vi "main.vi"() -> ()   [LabVIEW 2020]
uses:
  PCANBasic/eX/CTLs/TPCANHandle-Channel_eX.ctl
  PCANBasic/eX/CTLs/TPCANHandle-Bitrate_eX.ctl
  PCANBasic/eX/CTLs/CAN MSG_eX.ctl
  PCANBasic/eX/CTLs/CAN ErrorTypes_eX.ctl
  PCANBasic/PCANBasic_eX.lvlib
panel:
  out "error out":errorcluster
  out "Rotary Init REPONSE ?":bool
  in  "stop":bool
  in  "SetBrightness":bool
  in  "Brightness \n(0xFE = OFF, 0xFD=MAX)":u8=253 format="%02x"
  in  "TPCANHandle-Bitrate":T1=enum."500 KBit/s"
  in  "TPCANHandle-Channel":T2
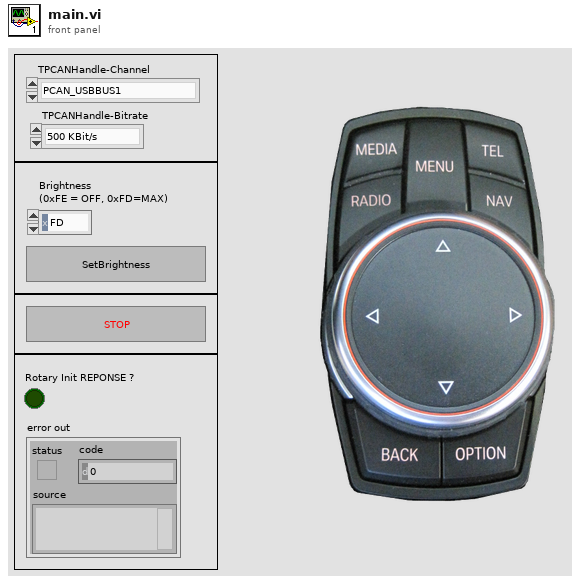
[diagram p1: front panel]
types:
  T1 = typedef "PCANBasic_eX.lvlib/TPCANHandle-Bitrate_eX.ctl" = enum16{"1 Mbit/s", "800 KBit/s", "500 KBit/s", "250 KBit/s", "125 KBit/s", "100 KBit/s"}
  T2 = typedef "PCANBasic_eX.lvlib/TPCANHandle-Channel_eX.ctl" = enum16{"PCAN_USBBUS1", "PCAN_USBBUS2"}
  T3 = typedef "PCANBasic_eX.lvlib/CAN MSG_eX.ctl" = cluster{"ID":u32, "MSGTYPE":u8, "LEN":u8, "DATA[0]":u8, "DATA[1]":u8, "DATA[2]":u8, "DATA[3]":u8, "DATA[4]":u8, "DATA[5]":u8, "DATA[6]":u8, "DATA[7]":u8}
  T4 = typedef "PCANBasic_eX.lvlib/CAN ErrorTypes_eX.ctl" = enum16{"ERROR_INIT", "ERROR_SEND_MSG", "ERROR_RECV_MSG", "ERROR_RESET", "ERROR_FILTER", "ERROR_UNINIT"}
  T5 = typedef "PCANBasic_eX.lvlib/CAN Timestamp_eX.ctl" = cluster{"millis":u32, "millis_overflow":u16, "micros":u16}
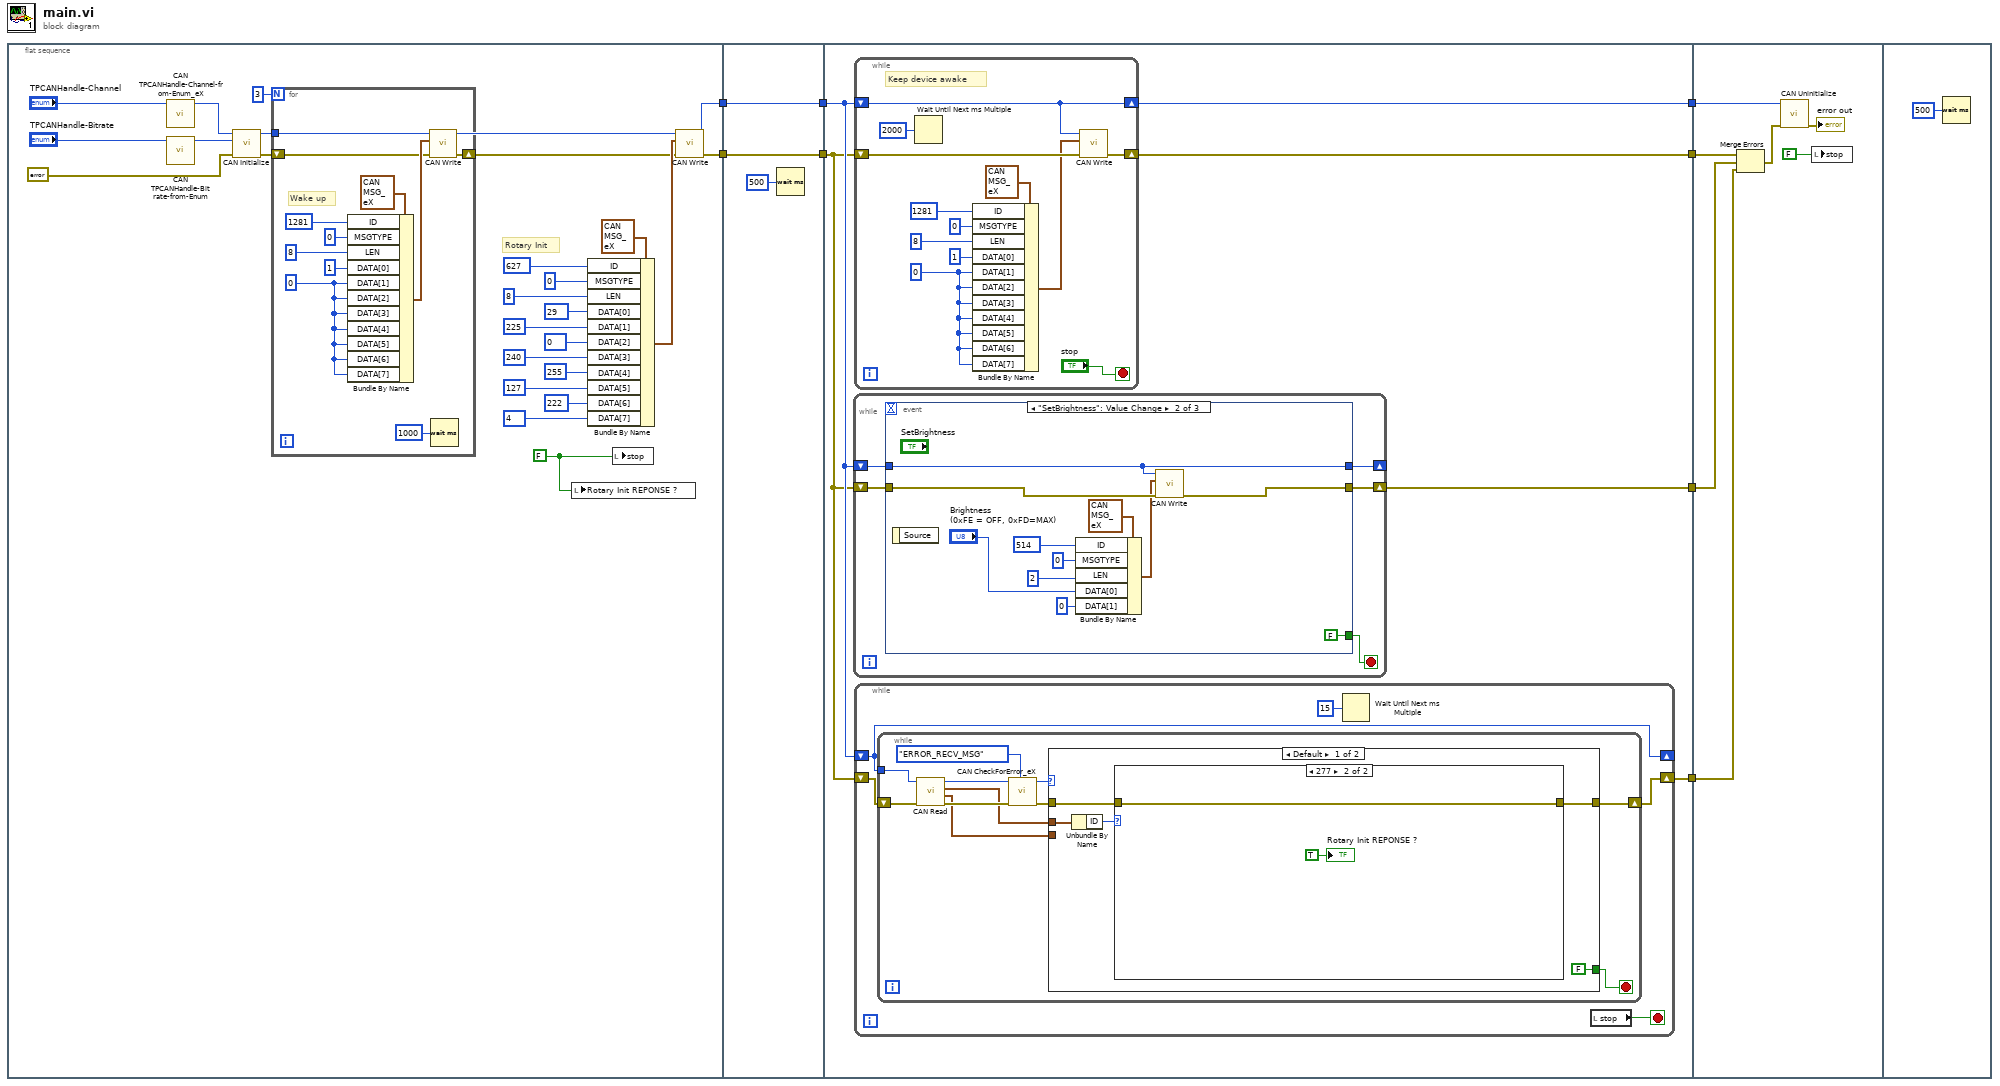
[diagram p0: block diagram]
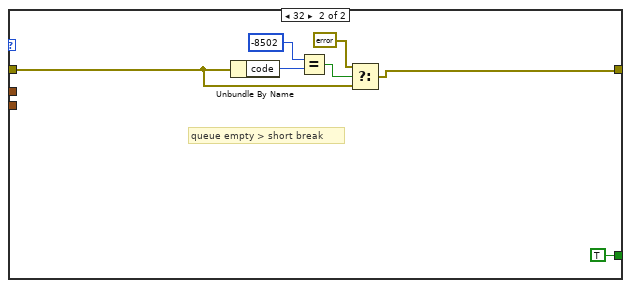
[diagram p3: hidden frame]
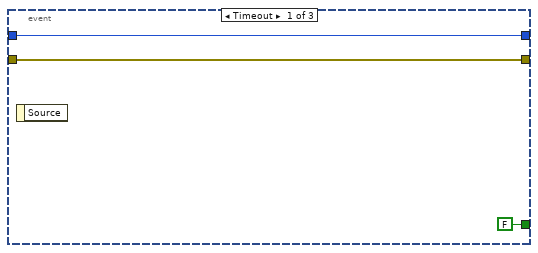
[diagram p4: hidden frame]
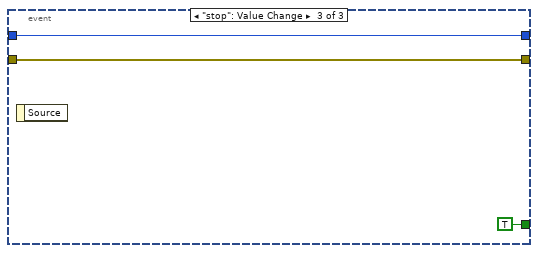
[diagram p5: hidden frame]
diagram:
  n1 = flat-sequence {
    tunnel: [w26] -> w8
    tunnel: [w25] -> w6
    tunnel: w8 -> [w45]
    tunnel: [w45] -> w7
    tunnel: w6 -> [w44]
    tunnel: [w44] -> w5
    tunnel: w7 -> [w50]
    tunnel: w5 -> [w51]
    tunnel: [w49] -> w4
    tunnel: [w48] -> w3
    tunnel: [w47] -> w2
    tunnel: [w46] -> w1
    tunnel: w4 -> [w123]
    tunnel: w3 -> [w122]
    tunnel: w2 -> [w121]
    tunnel: w1 -> [w119]
    frame #0 {
      w11 = FALSE ("stop")
      # "Rotary Init"
      n2 = call "CAN TPCANHandle-Channel-from-Enum_eX.vi"("TPCANHandle-Channel"="TPCANHandle-Channel") -> ("Channel"=w25:u16)  [unwired: 10 in]
      n3 = call "CAN TPCANHandle-Bitrate-from-Enum.vi"("TPCANHandle-Bitrate"="TPCANHandle-Bitrate") -> ("Btr0Btr1"=w31:u16)  [unwired: 10 in]
      n4 = call "CAN Initialize.vi"("error in (no error)"=errorcluster {"status"=FALSE, "code"=0, "source"=""}, "Btr0Btr1"=w31, "Channel"=w25) -> ("error out"=w27:errorcluster)  [unwired: 7 in, 1 out]
      n5 = for {
        N: 3 -> [_]
        tunnel: w25 -> [w34]
        shift-right: [w33] -> w10
        shift-left: w27 -> [w35]
        w42 = u8 0 ("DATA[1]")
        # "Wake up"
        n6 = Bundle By Name(cluster=T3 {"ID"=261, "MSGTYPE"=0, "LEN"=8, "DATA[0]"=37, "DATA[1]"=80, "DATA[2]"=37, "DATA[3]"=80, "DATA[4]"=37, "DATA[5]"=80, "DATA[6]"=37, "DATA[7]"=80} ("MessageBuffer"), "ID"=u32 1281, "MSGTYPE"=u8 0, "LEN"=u8 8, "DATA[0]"=u8 1, "DATA[1]"=w42, "DATA[2]"=w42, "DATA[3]"=w42, "DATA[4]"=w42, "DATA[5]"=w42, "DATA[6]"=w42, "DATA[7]"=w42) -> (w37:T3)
        n7 = call "CAN Write.vi"("error in (no error)"=w35, "MessageBuffer"=w37, "Channel"=w34) -> ("error out"=w33:errorcluster)  [unwired: 6 in, 2 out]
        n8 = Wait (ms)(milliseconds to wait=u32 1000) -> ()  [unwired: 1 out]
      }
      n9 = local write "Rotary Init REPONSE ?"(w11) -> ()
      n10 = Bundle By Name(cluster=T3 {"ID"=261, "MSGTYPE"=0, "LEN"=8, "DATA[0]"=37, "DATA[1]"=80, "DATA[2]"=37, "DATA[3]"=80, "DATA[4]"=37, "DATA[5]"=80, "DATA[6]"=37, "DATA[7]"=80} ("MessageBuffer"), "ID"=u32 627, "MSGTYPE"=u8 0, "LEN"=u8 8, "DATA[0]"=u8 29, "DATA[1]"=u8 225 ("DATA[0]"), "DATA[2]"=u8 0 ("DATA[0]"), "DATA[3]"=u8 240 ("DATA[0]"), "DATA[4]"=u8 255 ("DATA[0]"), "DATA[5]"=u8 127 ("DATA[0]"), "DATA[6]"=u8 222 ("DATA[0]"), "DATA[7]"=u8 4 ("DATA[0]")) -> (w20:T3)
      n11 = local write "stop"(w11) -> ()
      n12 = call "CAN Write.vi"("error in (no error)"=w10, "MessageBuffer"=w20, "Channel"=w25) -> ("error out"=w26:errorcluster)  [unwired: 6 in, 2 out]
    }
    frame #1 {
      n13 = Wait (ms)(milliseconds to wait=u32 500) -> ()  [unwired: 1 out]
    }
    frame #2 {
      n14 = while {
        shift-right: [w85] -> w48
        shift-left: w50 -> [w86]
        shift-right: [w84] -> _
        shift-left: w51 -> [w87]
        stop <- w83 stop-if-true
        n15 = event shown="[1] \"SetBrightness\": Value Change" {
          selector: _ -> [_ _ _]
          dyn-events: _ -> [_ _ _]
          timeout: _ -> [_ _ _]
          tunnel: w87 -> [w90 w92 w104]
          tunnel: w86 -> [w89 w101 w103]
          tunnel: [w89 w93 w103] -> w85
          tunnel: [w90 w92 w104] -> w84
          tunnel: [FALSE ("stop") FALSE ("stop") TRUE ("stop")] -> w83
          event Timeout {
            n16 = event-data() -> ()  [unwired: 1 in, 1 out]
          }
          event "SetBrightness": Value Change {
            n17 = event-data() -> ()  [unwired: 1 in, 1 out]
            n18 = Bundle By Name(cluster=T3 {"ID"=261, "MSGTYPE"=0, "LEN"=8, "DATA[0]"=37, "DATA[1]"=80, "DATA[2]"=37, "DATA[3]"=80, "DATA[4]"=37, "DATA[5]"=80, "DATA[6]"=37, "DATA[7]"=80} ("MessageBuffer"), "ID"=u32 514, "MSGTYPE"=u8 0, "LEN"=u8 2, "DATA[0]"="Brightness \n(0xFE = OFF, 0xFD=MAX)", "DATA[1]"=u8 0) -> (w98:T3)
            n19 = call "CAN Write.vi"("error in (no error)"=w101, "MessageBuffer"=w98, "Channel"=w92) -> ("error out"=w93:errorcluster)  [unwired: 6 in, 2 out]
          }
          event "stop": Value Change {
            n20 = event-data() -> ()  [unwired: 1 in, 1 out]
          }
        }
      }
      n21 = while {
        shift-right: [w106] -> w49
        shift-left: w50 -> [w115]
        shift-right: [w107] -> w46
        shift-left: w51 -> [w107]
        stop <- "stop" stop-if-true
        w108 = u8 0 ("DATA[1]")
        # "Keep device awake"
        n22 = Wait Until Next ms Multiple(millisecond multiple=u32 2000) -> ()  [unwired: 1 out]
        n23 = Bundle By Name(cluster=T3 {"ID"=261, "MSGTYPE"=0, "LEN"=8, "DATA[0]"=37, "DATA[1]"=80, "DATA[2]"=37, "DATA[3]"=80, "DATA[4]"=37, "DATA[5]"=80, "DATA[6]"=37, "DATA[7]"=80} ("MessageBuffer"), "ID"=u32 1281, "MSGTYPE"=u8 0, "LEN"=u8 8, "DATA[0]"=u8 1, "DATA[1]"=w108, "DATA[2]"=w108, "DATA[3]"=w108, "DATA[4]"=w108, "DATA[5]"=w108, "DATA[6]"=w108, "DATA[7]"=w108) -> (w113:T3)
        n24 = call "CAN Write.vi"("error in (no error)"=w115, "MessageBuffer"=w113, "Channel"=w107) -> ("error out"=w106:errorcluster)  [unwired: 6 in, 2 out]
      }
      n25 = while {
        shift-right: [w53] -> w47
        shift-left: w50 -> [w55]
        shift-right: [w54] -> _
        shift-left: w51 -> [w54]
        stop <- w52 stop-if-true
        n26 = while {
          tunnel: w54 -> [w67]
          shift-right: [w60] -> w53
          shift-left: w55 -> [w66]
          stop <- w59 stop-if-true
          n27 = call "CAN Read.vi"("error in (no error)"=w66, "Channel"=w67) -> ("error out"=w62:errorcluster, "TimestampBuffer out"=w57:T5, "MessageBuffer out"=w58:T3, "function return"=w65:u32)  [unwired: 6 in]
          n28 = call "CAN CheckForError_eX.vi"("ErrorType"=CAN_ErrorTypes_eX."ERROR_RECV_MSG", "error in (no error)"=w62, "TPCANStatus"=w65) -> ("error out"=w61:errorcluster, "TPCANStatus out"=w63:u32)  [unwired: 7 in]
          n29 = case shown="Default" w63 {
            tunnel: w61 -> [w68 w78]
            tunnel: [w69 w77] -> w60
            tunnel: [FALSE TRUE] -> w59
            tunnel: w58 -> [w71 _]
            tunnel: w57 -> [_ _]
            frame Default {
              n30 = Unbundle By Name(w71) -> ("ID"=w70:u32)
              n31 = case shown="277" w70 {
                tunnel: [w73 w75] -> w69
                tunnel: w68 -> [w73 w75]
                frame Default {
                }
                frame 631 {
                  "Rotary Init REPONSE ?" <- TRUE ("Rotary Init REPONSE ?")
                }
              }
            }
            frame 32 {
              # "queue empty > short break"
              n32 = Unbundle By Name(w78) -> ("code"=w80:i32)
              n33 = Equal?(x=-8502, y=w80) -> (x = y?=w81:bool)
              n34 = Select(t=errorcluster {"status"=FALSE, "code"=0, "source"=""} ("error constant"), s=w81, f=w78) -> (s? t:f=w77:errorcluster)
            }
          }
        }
        n35 = Wait Until Next ms Multiple(millisecond multiple=u32 15) -> ()  [unwired: 1 out]
        n36 = local read "stop"() -> (w52:bool)
      }
    }
    frame #3 {
      n37 = Merge Errors(w123, w122, w121) -> (w120:errorcluster)
      n38 = call "CAN Uninitialize.vi"("error in (no error)"=w120, "Channel"=w119) -> ("error out"=→"error out":errorcluster)  [unwired: 8 in, 1 out]
      n39 = local write "stop"(FALSE ("stop")) -> ()
    }
    frame #4 {
      n40 = Wait (ms)(milliseconds to wait=u32 500) -> ()  [unwired: 1 out]
    }
  }
